vi "record_instr_data_window.vi"() -> ()   [LabVIEW 2013]
doc: "displays and records data from an Instrument (PreLineObject)"
uses:
  Classes/Instrument/instrument.lvclass
  Classes/PrepLineObject/PrepLineObject.lvclass
panel:
  out "current value 2":dbl format="%#_4g"
  out "current value 1":dbl format="%#_4g"
  in  "clear plot 2":bool
  in  "clear plot 1":bool
  out "found InstrObject 2":refnum<class "instrument.lvclass">
  out "found PrepLineObject 2":refnum<class "PrepLineObject.lvclass">
  out "name2_valid?":bool
  out "name1_valid?":bool
  out "XY Graph 2":cluster{"X":dbl, "Y":dbl}[](graph)
  out "close?":bool
  out "found PrepLineObject 1":refnum<class "PrepLineObject.lvclass">
  out "found InstrObject 1":refnum<class "instrument.lvclass">
  in  "sampling time [s]":u32
  in  "record button":bool
  in  "Listbox":i32(listbox)
  out "XY Graph":cluster{"X":dbl, "Y":dbl}[](graph)
  # "drag and drop item into plot"
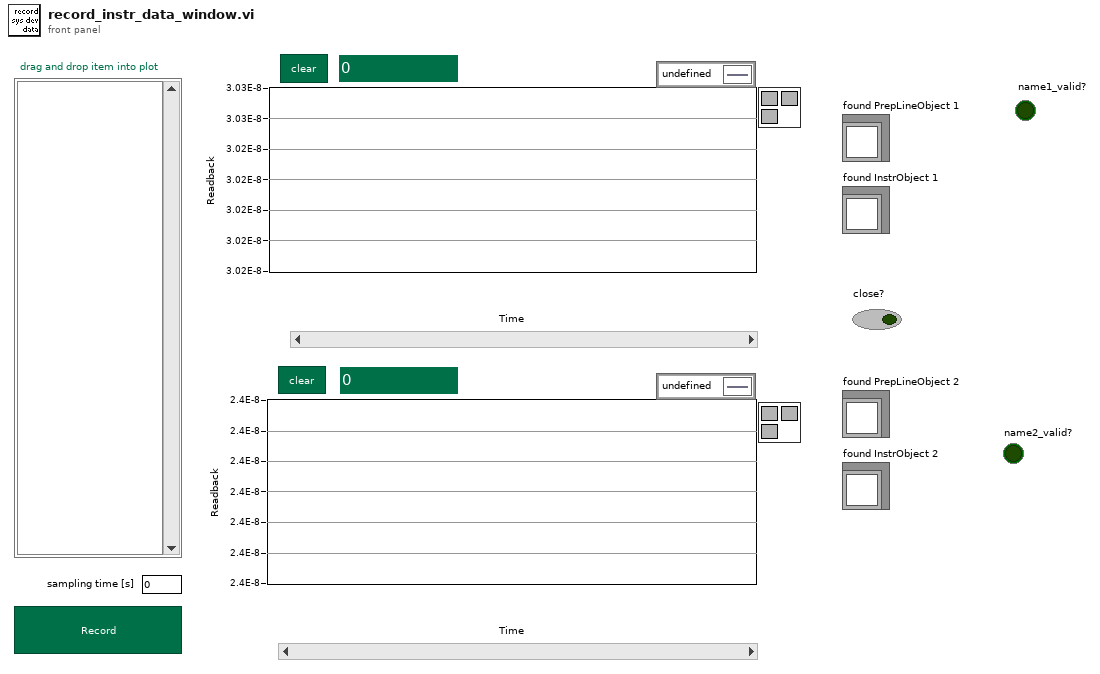
[diagram p1: front panel]
types:
  T1 = enum8{"Enabled", "Disabled", "Disabled and Grayed Out"}
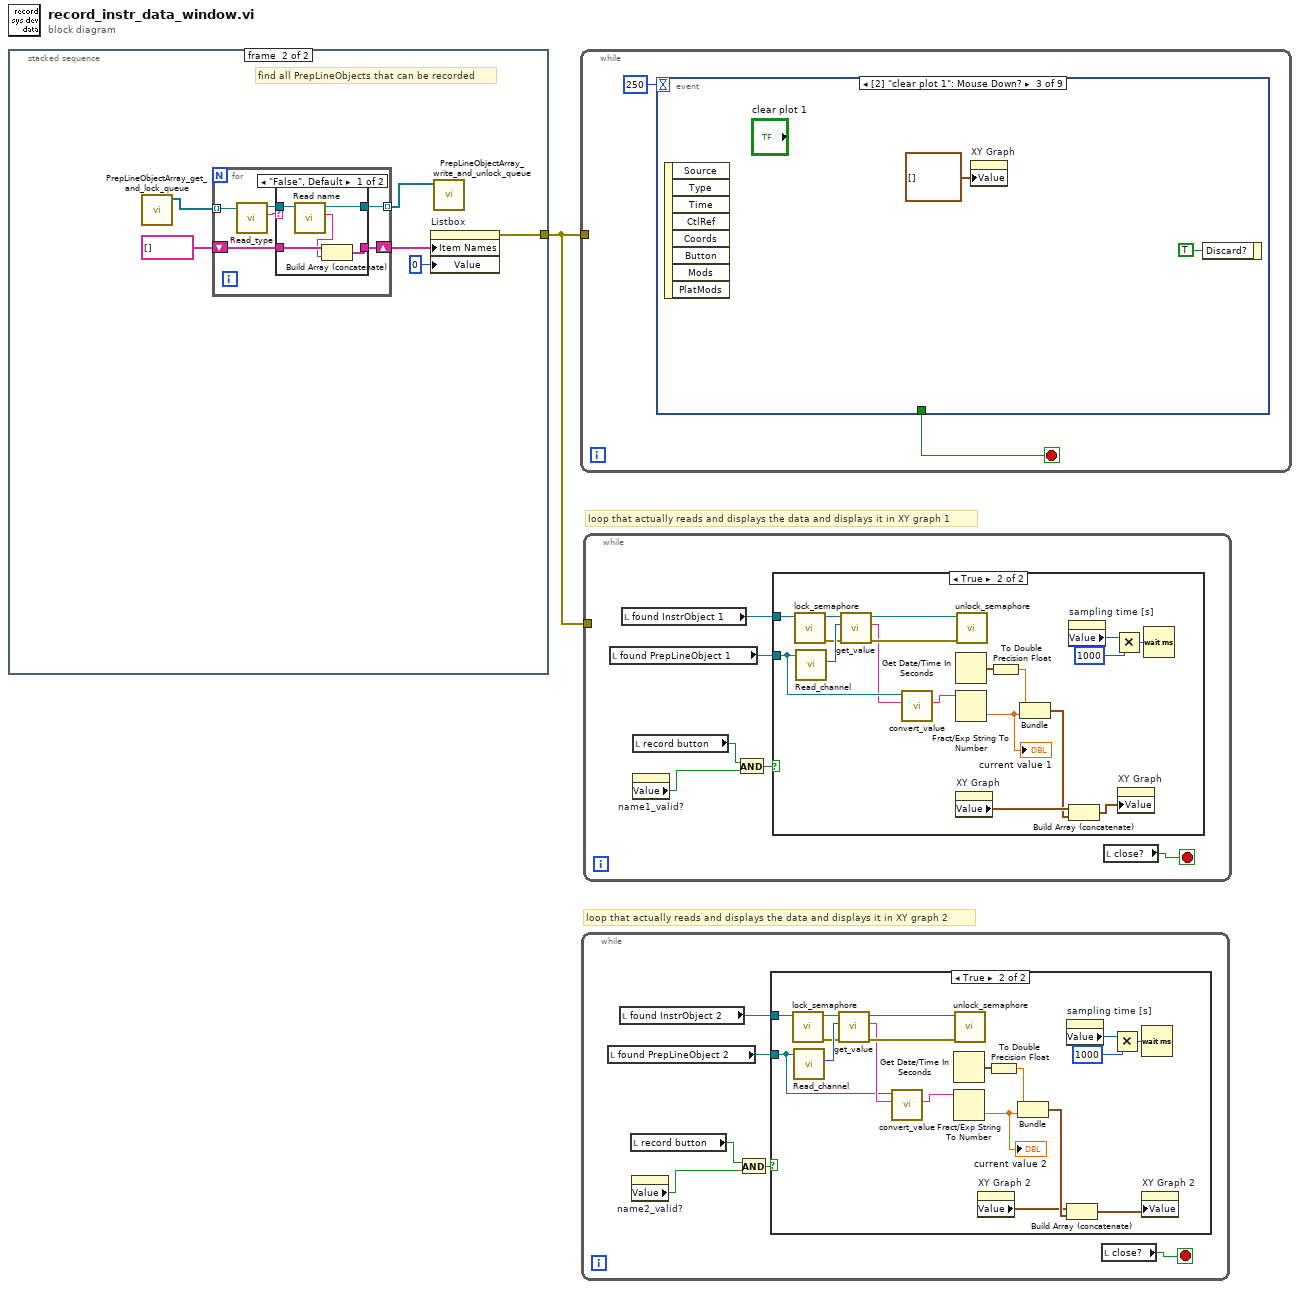
[diagram p0: block diagram]
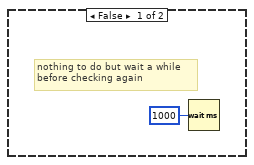
[diagram p2: hidden frame]
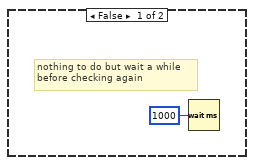
[diagram p3: hidden frame]
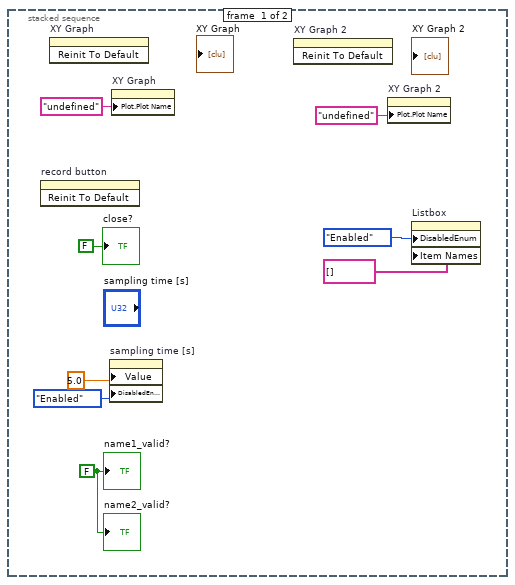
[diagram p4: hidden frame]
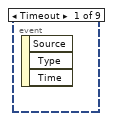
[diagram p6: hidden frame]
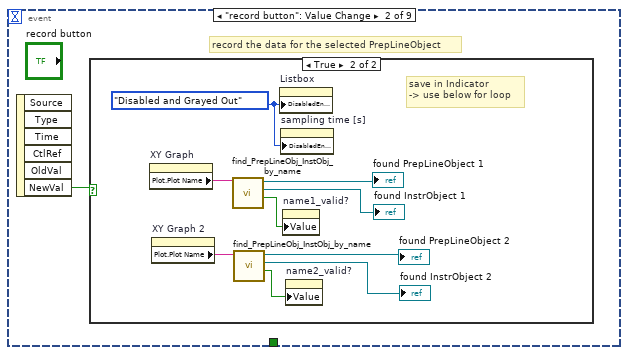
[diagram p7: hidden frame]
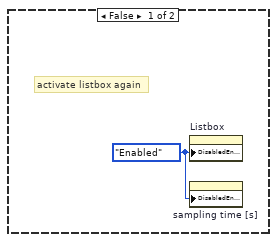
[diagram p8: hidden frame]
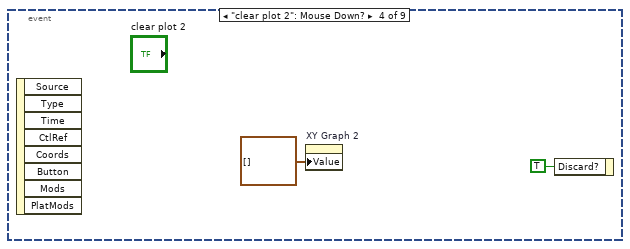
[diagram p9: hidden frame]
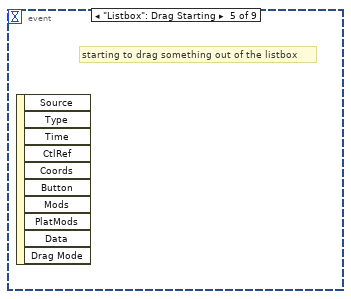
[diagram p10: hidden frame]
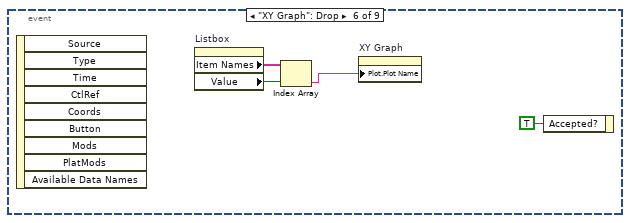
[diagram p11: hidden frame]
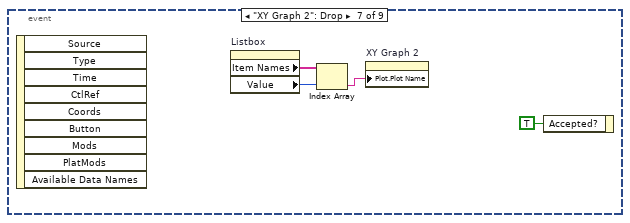
[diagram p12: hidden frame]
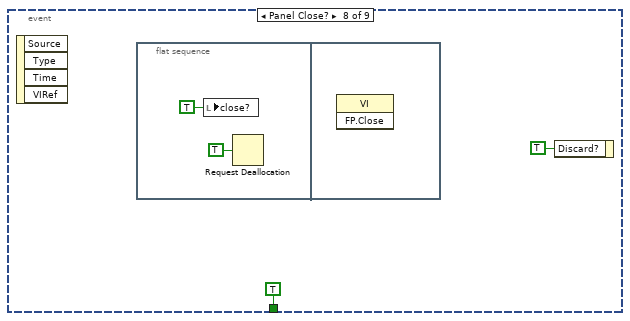
[diagram p13: hidden frame]
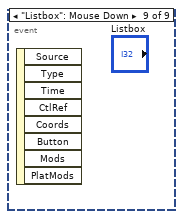
[diagram p14: hidden frame]
diagram:
  # "loop that actually reads and displays the data and displays it in XY graph 2"
  # "loop that actually reads and displays the data and displays it in XY graph 1"
  n1 = stacked-sequence {
    tunnel: [_ w12] -> w1
    frame #0 {
      w3 = FALSE ("name1 valid?")
      n2 = invoke on="record button" class="Bool (strict)" method="Reinit To Default"() -> ()  [unwired: 3 in, 3 out]
      n3 = invoke on="XY Graph" class="XYGraph (strict)" method="Reinit To Default"() -> ()  [unwired: 3 in, 3 out]
      n4 = property on="sampling time [s]" class="DigNum (strict)"("Value"=5.0 ("sampling time [s]"), "DisabledEnum"=T1."Enabled" ("Disabled")) -> ()  [unwired: 2 in, 2 out]
      n5 = property on="XY Graph" class="XYGraph (strict)"("Plot.Plot Name"="undefined") -> ()  [unwired: 2 in, 2 out]
      n6 = invoke on="XY Graph 2" class="XYGraph (strict)" method="Reinit To Default"() -> ()  [unwired: 3 in, 3 out]
      n7 = property on="XY Graph 2" class="XYGraph (strict)"("Plot.Plot Name"="undefined") -> ()  [unwired: 2 in, 2 out]
      n8 = property on="Listbox" class="LstBox (strict)"("DisabledEnum"=T1."Enabled" ("Disabled"), "Item Names"=string[] []) -> ()  [unwired: 2 in, 2 out]
      "close?" <- FALSE ("close?")
      "name1_valid?" <- w3
      "name2_valid?" <- w3
    }
    frame #1 {
      # "find all PrepLineObjects that can be recorded"
      n9 = call "PrepLineObjectArray_get_and_lock_queue.vi"() -> ("PrepLineObjects"=w11:refnum<class "PrepLineObject.lvclass">[])  [unwired: 10 in, 1 out]
      n10 = for {
        tunnel: w11 -> [w21] mode=indexing
        shift-right: [w17] -> w14
        shift-left: string[] [] -> [w18]
        tunnel: [w16] -> w10 mode=indexing
        n11 = call-dynamic "Read_type.vi"("PrepLinePictureObjects in"=w21) -> ("String"=w20:string, "PrepLinePictureObjects out"=w19:refnum<class "PrepLineObject.lvclass">)  [unwired: 8 in, 1 out]
        n12 = case shown="\"False\", Default" w20 {
          tunnel: w19 -> [w26 w27]
          tunnel: w18 -> [w25 w28]
          tunnel: [w24 w28] -> w17
          tunnel: [w22 w27] -> w16
          frame "False", Default {
            n13 = call-dynamic "Read name.vi"("PrepLineObject in"=w26) -> ("name"=w23:string, "PrepLineObject out"=w22:refnum<class "PrepLineObject.lvclass">)  [unwired: 8 in, 1 out]
            n14 = Build Array (concatenate)(w25, w23) -> (w24:string[])
          }
          frame "switch" {
          }
        }
      }
      n15 = property on="Listbox" class="LstBox (strict)"("Item Names"=w14, "Value"=0 ("Listbox")) -> (error out=w12:errorcluster)  [unwired: 2 in, 1 out]
      n16 = call "PrepLineObjectArray_write_and_unlock_queue.vi"("PrepLineObjArray"=w10) -> ()  [unwired: 10 in, 1 out]
    }
  }
  n17 = while {
    tunnel: w1 -> [_]
    stop <- w30 stop-if-true
    n18 = event shown="[2] \"clear plot 1\": Mouse Down?" {
      selector: _ -> [_ _ _ _ _ _ _ _ _]
      dyn-events: _ -> [_ _ _ _ _ _ _ _ _]
      timeout: 250 -> [_ _ _ _ _ _ _ _ _]
      tunnel: [_ _ _ _ _ _ _ TRUE _] -> w30
      event Timeout {
        n19 = event-data() -> ()  [unwired: 1 in, 3 out]
      }
      event "record button": Value Change {
        # "record the data for the selected PrepLineObject"
        n20 = event-data() -> ("NewVal"=w31:bool)  [unwired: 1 in, 5 out]
        n21 = case shown="True" w31 {
          frame False {
            w32 = T1."Enabled" ("Disabled")
            # "activate listbox again"
            n22 = property on="Listbox" class="LstBox (strict)"("DisabledEnum"=w32) -> ()  [unwired: 2 in, 2 out]
            n23 = property on="sampling time [s]" class="DigNum (strict)"("DisabledEnum"=w32) -> ()  [unwired: 2 in, 2 out]
          }
          frame True {
            w33 = T1."Disabled and Grayed Out" ("Disabled")
            # "save in Indicator\n-> use below for loop"
            n24 = property on="XY Graph" class="XYGraph (strict)"() -> ("Plot.Plot Name"=w41:string)  [unwired: 2 in, 2 out]
            n25 = property on="XY Graph 2" class="XYGraph (strict)"() -> ("Plot.Plot Name"=w35:string)  [unwired: 2 in, 2 out]
            n26 = call "find_PrepLineObj_InstObj_by_name.vi"("PrepLineObject Name"=w41) -> ("found?"=w38:bool, "found InstrObject out"=→"found InstrObject 1":refnum<class "instrument.lvclass">, "found PrepLineObject out"=→"found PrepLineObject 1":refnum<class "PrepLineObject.lvclass">)  [unwired: 7 in, 1 out]
            n27 = call "find_PrepLineObj_InstObj_by_name.vi"("PrepLineObject Name"=w35) -> ("found?"=w34:bool, "found InstrObject out"=→"found InstrObject 2":refnum<class "instrument.lvclass">, "found PrepLineObject out"=→"found PrepLineObject 2":refnum<class "PrepLineObject.lvclass">)  [unwired: 7 in, 1 out]
            n28 = property on="Listbox" class="LstBox (strict)"("DisabledEnum"=w33) -> ()  [unwired: 2 in, 2 out]
            n29 = property on="sampling time [s]" class="DigNum (strict)"("DisabledEnum"=w33) -> ()  [unwired: 2 in, 2 out]
            n30 = property on="name1_valid?" class="Bool (strict)"("Value"=w38) -> ()  [unwired: 2 in, 2 out]
            n31 = property on="name2_valid?" class="Bool (strict)"("Value"=w34) -> ()  [unwired: 2 in, 2 out]
          }
        }
      }
      event "clear plot 1": Mouse Down? {
        n32 = event-data() -> ()  [unwired: 1 in, 8 out]
        n33 = property on="XY Graph" class="XYGraph (strict)"("Value"=cluster{"X":dbl, "Y":dbl}[] [] ("XY Graph")) -> ()  [unwired: 2 in, 2 out]
        n34 = event-data("Discard?"=TRUE) -> ()  [unwired: 1 in, 1 out]
      }
      event "clear plot 2": Mouse Down? {
        n35 = event-data() -> ()  [unwired: 1 in, 8 out]
        n36 = property on="XY Graph 2" class="XYGraph (strict)"("Value"=cluster{"X":dbl, "Y":dbl}[] [] ("XY Graph 2")) -> ()  [unwired: 2 in, 2 out]
        n37 = event-data("Discard?"=TRUE) -> ()  [unwired: 1 in, 1 out]
      }
      event "Listbox": Drag Starting {
        # "starting to drag something out of the listbox"
        n38 = event-data() -> ()  [unwired: 1 in, 10 out]
      }
      event "XY Graph": Drop {
        n39 = event-data() -> ()  [unwired: 1 in, 9 out]
        n40 = property on="Listbox" class="LstBox (strict)"() -> ("Item Names"=w48:string[], "Value"=w49:i32)  [unwired: 2 in, 2 out]
        n41 = Index Array(array=w48, index=w49) -> (element=w47:string)
        n42 = property on="XY Graph" class="XYGraph (strict)"("Plot.Plot Name"=w47) -> ()  [unwired: 2 in, 2 out]
        n43 = event-data("Accepted?"=TRUE) -> ()  [unwired: 1 in, 1 out]
      }
      event "XY Graph 2": Drop {
        n44 = event-data() -> ()  [unwired: 1 in, 9 out]
        n45 = property on="Listbox" class="LstBox (strict)"() -> ("Item Names"=w52:string[], "Value"=w53:i32)  [unwired: 2 in, 2 out]
        n46 = Index Array(array=w52, index=w53) -> (element=w51:string)
        n47 = property on="XY Graph 2" class="XYGraph (strict)"("Plot.Plot Name"=w51) -> ()  [unwired: 2 in, 2 out]
        n48 = event-data("Accepted?"=TRUE) -> ()  [unwired: 1 in, 1 out]
      }
      event Panel Close? {
        n49 = event-data() -> ()  [unwired: 1 in, 4 out]
        n50 = flat-sequence {
          frame #0 {
            n51 = local write "close?"(TRUE ("close?")) -> ()
            n52 = Request Deallocation(TRUE ("flag")) -> ()
          }
          frame #1 {
            n53 = invoke class="VI" method="FP.Close"() -> ()  [unwired: 3 in, 3 out]
          }
        }
        n54 = event-data("Discard?"=TRUE) -> ()  [unwired: 1 in, 1 out]
      }
      event "Listbox": Mouse Down {
        n55 = event-data() -> ()  [unwired: 1 in, 8 out]
      }
    }
  }
  n56 = while {
    stop <- w63 stop-if-true
    n57 = local read "found PrepLineObject 2"() -> (w61:refnum<class "PrepLineObject.lvclass">)
    n58 = local read "found InstrObject 2"() -> (w62:refnum<class "instrument.lvclass">)
    n59 = local read "record button"() -> (w60:bool)
    n60 = property on="name2_valid?" class="Bool (strict)"() -> ("Value"=w58:bool)  [unwired: 2 in, 2 out]
    n61 = And(x=w60, y=w58) -> (x .and. y?=w59:bool)
    n62 = case shown="True" w59 {
      tunnel: w62 -> [_ w76]
      tunnel: w61 -> [_ w65]
      frame False {
        # "nothing to do but wait a while\nbefore checking again"
        n63 = Wait (ms)(milliseconds to wait=u32 1000) -> ()  [unwired: 1 out]
      }
      frame True {
        n64 = call-dynamic "lock_semaphore.vi"("instrument in"=w76) -> ("error out"=w79:errorcluster, "instrument out"=w80:refnum<class "instrument.lvclass">)  [unwired: 9 in]
        n65 = call-dynamic "Read_channel.vi"("PrepLineObject in"=w65) -> ("channel"=w81:u16)  [unwired: 8 in, 2 out]
        n66 = call-dynamic "get_value.vi"("error in (no error)"=w79, "channel"=w81, "instrument in"=w80) -> ("error out"=w77:errorcluster, "value"=w67:string, "instrument out"=w78:refnum<class "instrument.lvclass">)  [unwired: 6 in]
        n67 = call-dynamic "convert_value.vi"("value in"=w67, "PrepLineObject in"=w65) -> ("converted value out"=w66:string)  [unwired: 7 in, 2 out]
        n68 = Get Date/Time In Seconds() -> (seconds since 1Jan1904=w82:timestamp)
        n69 = Fract/Exp String To Number(string=w66) -> (number=w68:dbl)  [unwired: 3 in, 1 out]
        "current value 2" <- w68
        n70 = call-dynamic "unlock_semaphore.vi"("error in (no error)"=w77, "instrument in"=w78) -> ()  [unwired: 8 in, 2 out]
        n71 = property on="XY Graph 2" class="XYGraph (strict)"() -> ("Value"=w70:cluster{"X":dbl, "Y":dbl}[])  [unwired: 2 in, 2 out]
        n72 = To Double Precision Float(number=w82) -> (double precision float=w75:dbl)
        n73 = Bundle(w75, w68) -> (w74:cluster{dbl, dbl})  [unwired: 1 in]
        n74 = property on="sampling time [s]" class="DigNum (strict)"() -> ("Value"=w73:u32)  [unwired: 2 in, 2 out]
        n75 = Build Array (concatenate)(w70, w74) -> (w69:cluster{"X":dbl, "Y":dbl}[])
        n76 = Multiply(x=w73, y=u32 1000) -> (x*y=w72:u32)
        n77 = Wait (ms)(milliseconds to wait=w72) -> ()  [unwired: 1 out]
        n78 = property on="XY Graph 2" class="XYGraph (strict)"("Value"=w69) -> ()  [unwired: 2 in, 2 out]
      }
    }
    n79 = local read "close?"() -> (w63:bool)
  }
  n80 = while {
    tunnel: w1 -> [_]
    stop <- w88 stop-if-true
    n81 = local read "found PrepLineObject 1"() -> (w86:refnum<class "PrepLineObject.lvclass">)
    n82 = local read "found InstrObject 1"() -> (w87:refnum<class "instrument.lvclass">)
    n83 = local read "record button"() -> (w84:bool)
    n84 = property on="name1_valid?" class="Bool (strict)"() -> ("Value"=w83:bool)  [unwired: 2 in, 2 out]
    n85 = And(x=w84, y=w83) -> (x .and. y?=w85:bool)
    n86 = case shown="True" w85 {
      tunnel: w87 -> [_ w101]
      tunnel: w86 -> [_ w92]
      frame False {
        # "nothing to do but wait a while\nbefore checking again"
        n87 = Wait (ms)(milliseconds to wait=u32 1000) -> ()  [unwired: 1 out]
      }
      frame True {
        n88 = call-dynamic "lock_semaphore.vi"("instrument in"=w101) -> ("error out"=w104:errorcluster, "instrument out"=w105:refnum<class "instrument.lvclass">)  [unwired: 9 in]
        n89 = call-dynamic "Read_channel.vi"("PrepLineObject in"=w92) -> ("channel"=w106:u16)  [unwired: 8 in, 2 out]
        n90 = call-dynamic "get_value.vi"("error in (no error)"=w104, "channel"=w106, "instrument in"=w105) -> ("error out"=w102:errorcluster, "value"=w91:string, "instrument out"=w103:refnum<class "instrument.lvclass">)  [unwired: 6 in]
        n91 = call-dynamic "convert_value.vi"("value in"=w91, "PrepLineObject in"=w92) -> ("converted value out"=w90:string)  [unwired: 7 in, 2 out]
        n92 = Get Date/Time In Seconds() -> (seconds since 1Jan1904=w107:timestamp)
        n93 = Fract/Exp String To Number(string=w90) -> (number=w93:dbl)  [unwired: 3 in, 1 out]
        "current value 1" <- w93
        n94 = property on="XY Graph" class="XYGraph (strict)"() -> ("Value"=w99:cluster{"X":dbl, "Y":dbl}[])  [unwired: 2 in, 2 out]
        n95 = call-dynamic "unlock_semaphore.vi"("error in (no error)"=w102, "instrument in"=w103) -> ()  [unwired: 8 in, 2 out]
        n96 = To Double Precision Float(number=w107) -> (double precision float=w100:dbl)
        n97 = Bundle(w100, w93) -> (w98:cluster{dbl, dbl})  [unwired: 1 in]
        n98 = property on="sampling time [s]" class="DigNum (strict)"() -> ("Value"=w96:u32)  [unwired: 2 in, 2 out]
        n99 = Build Array (concatenate)(w99, w98) -> (w97:cluster{"X":dbl, "Y":dbl}[])
        n100 = Multiply(x=w96, y=u32 1000) -> (x*y=w95:u32)
        n101 = property on="XY Graph" class="XYGraph (strict)"("Value"=w97) -> ()  [unwired: 2 in, 2 out]
        n102 = Wait (ms)(milliseconds to wait=w95) -> ()  [unwired: 1 out]
      }
    }
    n103 = local read "close?"() -> (w88:bool)
  }
